vi "HILMarineTurbine.vi"() -> ()   [LabVIEW 2021]
uses:
  <vilib>/Utility/error.llb/DialogType.ctl
  <vilib>/DAQmx/read.llb/DAQmx Read (Analog 1D Wfm NChan NSamp).vi
  <vilib>/DAQmx/write.llb/DAQmx Write (Counter Frequency 1Chan 1Samp).vi
  <vilib>/Utility/file.llb/Read Delimited Spreadsheet (DBL).vi
  <vilib>/DAQmx/create/channels.llb/DAQmx Create Channel (CO-Pulse Generation-Frequency).vi
  <vilib>/DAQmx/configure/timing.llb/DAQmx Timing (Implicit).vi
  <vilib>/DAQmx/miscellaneous.llb/DAQmx Fill In Error Info.vi
  <vilib>/addons/control/pid/pid.llb/PID (DBL).vi
  <vilib>/addons/control/pid/NI_PID_pid.lvlib
panel:
  out "Waveform Graph 2":dynamicdata(graph)
  out "Waveform Graph":dynamicdata(graph)
  in  "Stop":bool
  out "XY Graph":cluster{"all rows":dbl[], "all rows":dbl[]}[](graph)
  out "Tm Turbina [Nm]":dbl
  out "Pm Turbina [W]":dbl
  in  "B [°]":dbl
  in  "Vf [m/s]":dbl
  out "Tm [Nm]":dbl
  out "Wm [RPM]":dbl
  out "P [W]":dbl
  out "IC [A]":dbl
  out "IB [A]":dbl
  out "IA [A]":dbl
  out "VCA [V]":dbl
  out "VBC [V]":dbl
  out "f [Hz] [Hz]":dbl
  out "VAB [V]":dbl
  # "Emulador de turbina marina"
  # "Voltaje"
  # "Corriente"
  # "Modelo matemático"
  # "Mediciones"
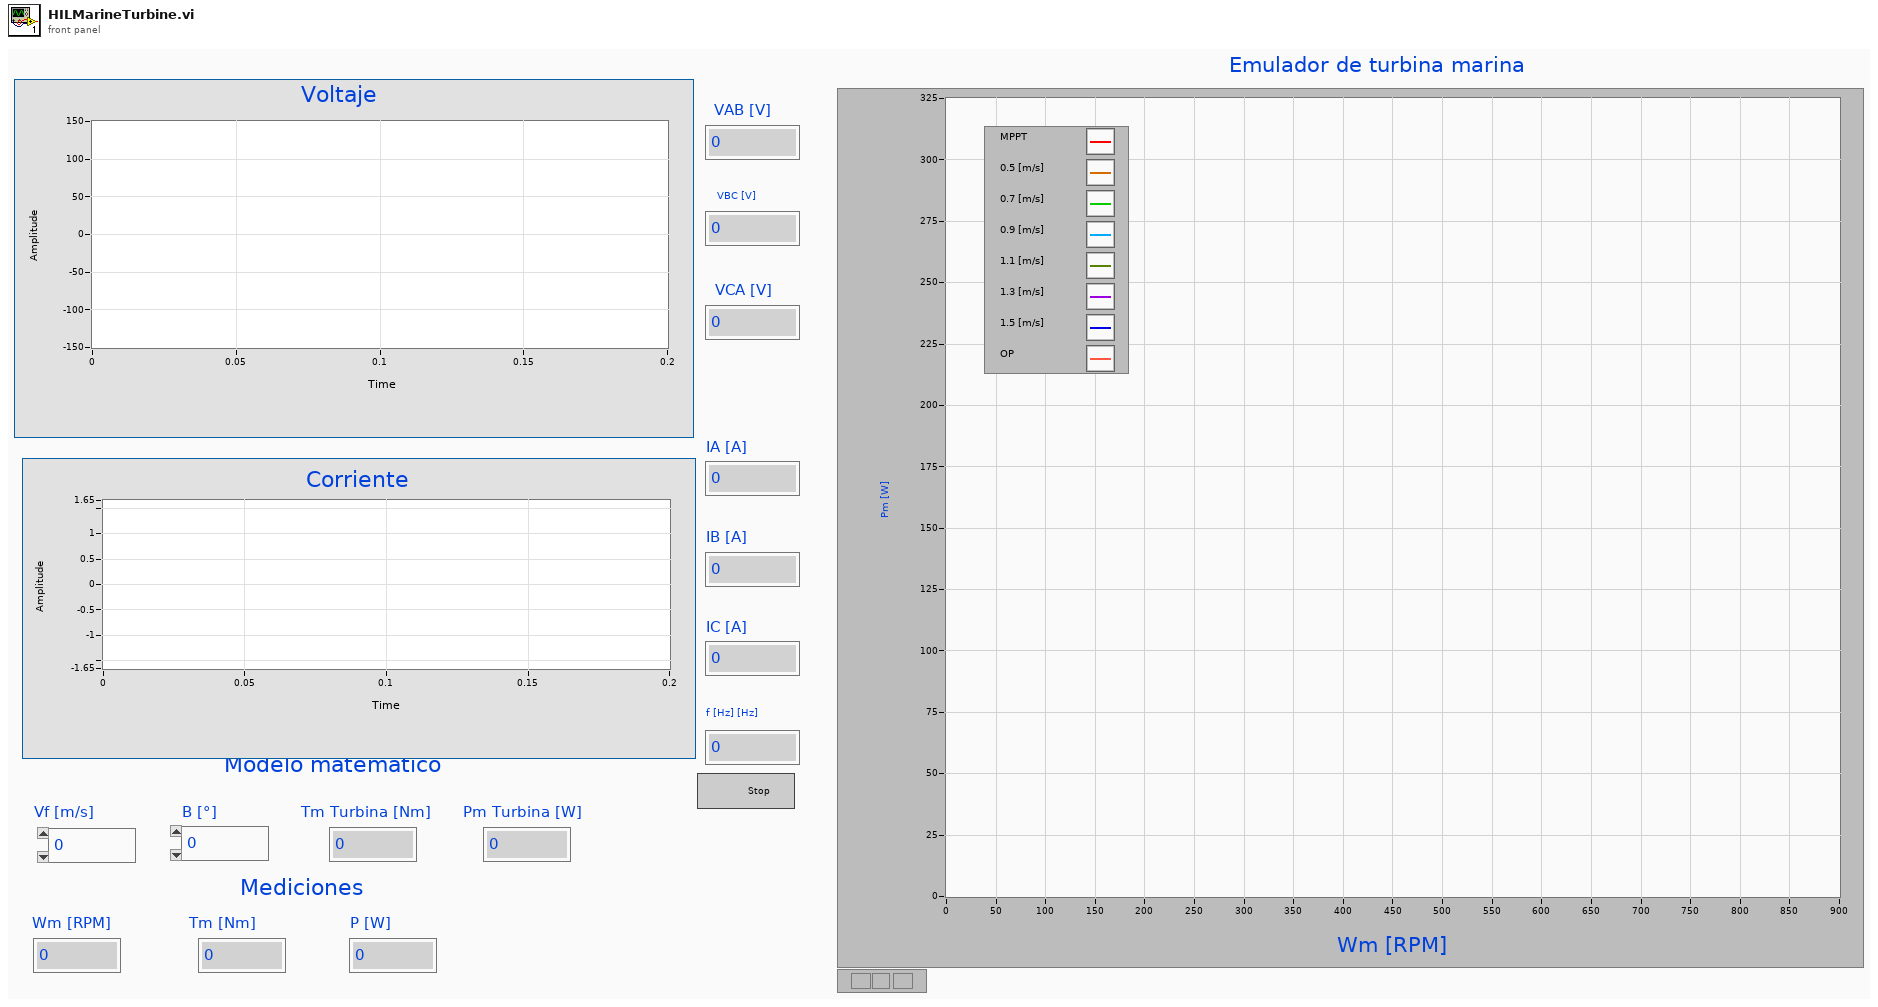
[diagram p1: front panel]
types:
  T1 = typedef "DialogType.ctl" = u16
  T2 = cluster{"proportional gain (Kc)":dbl, "integral time (Ti, min)":dbl, "derivative time (Td, min)":dbl}
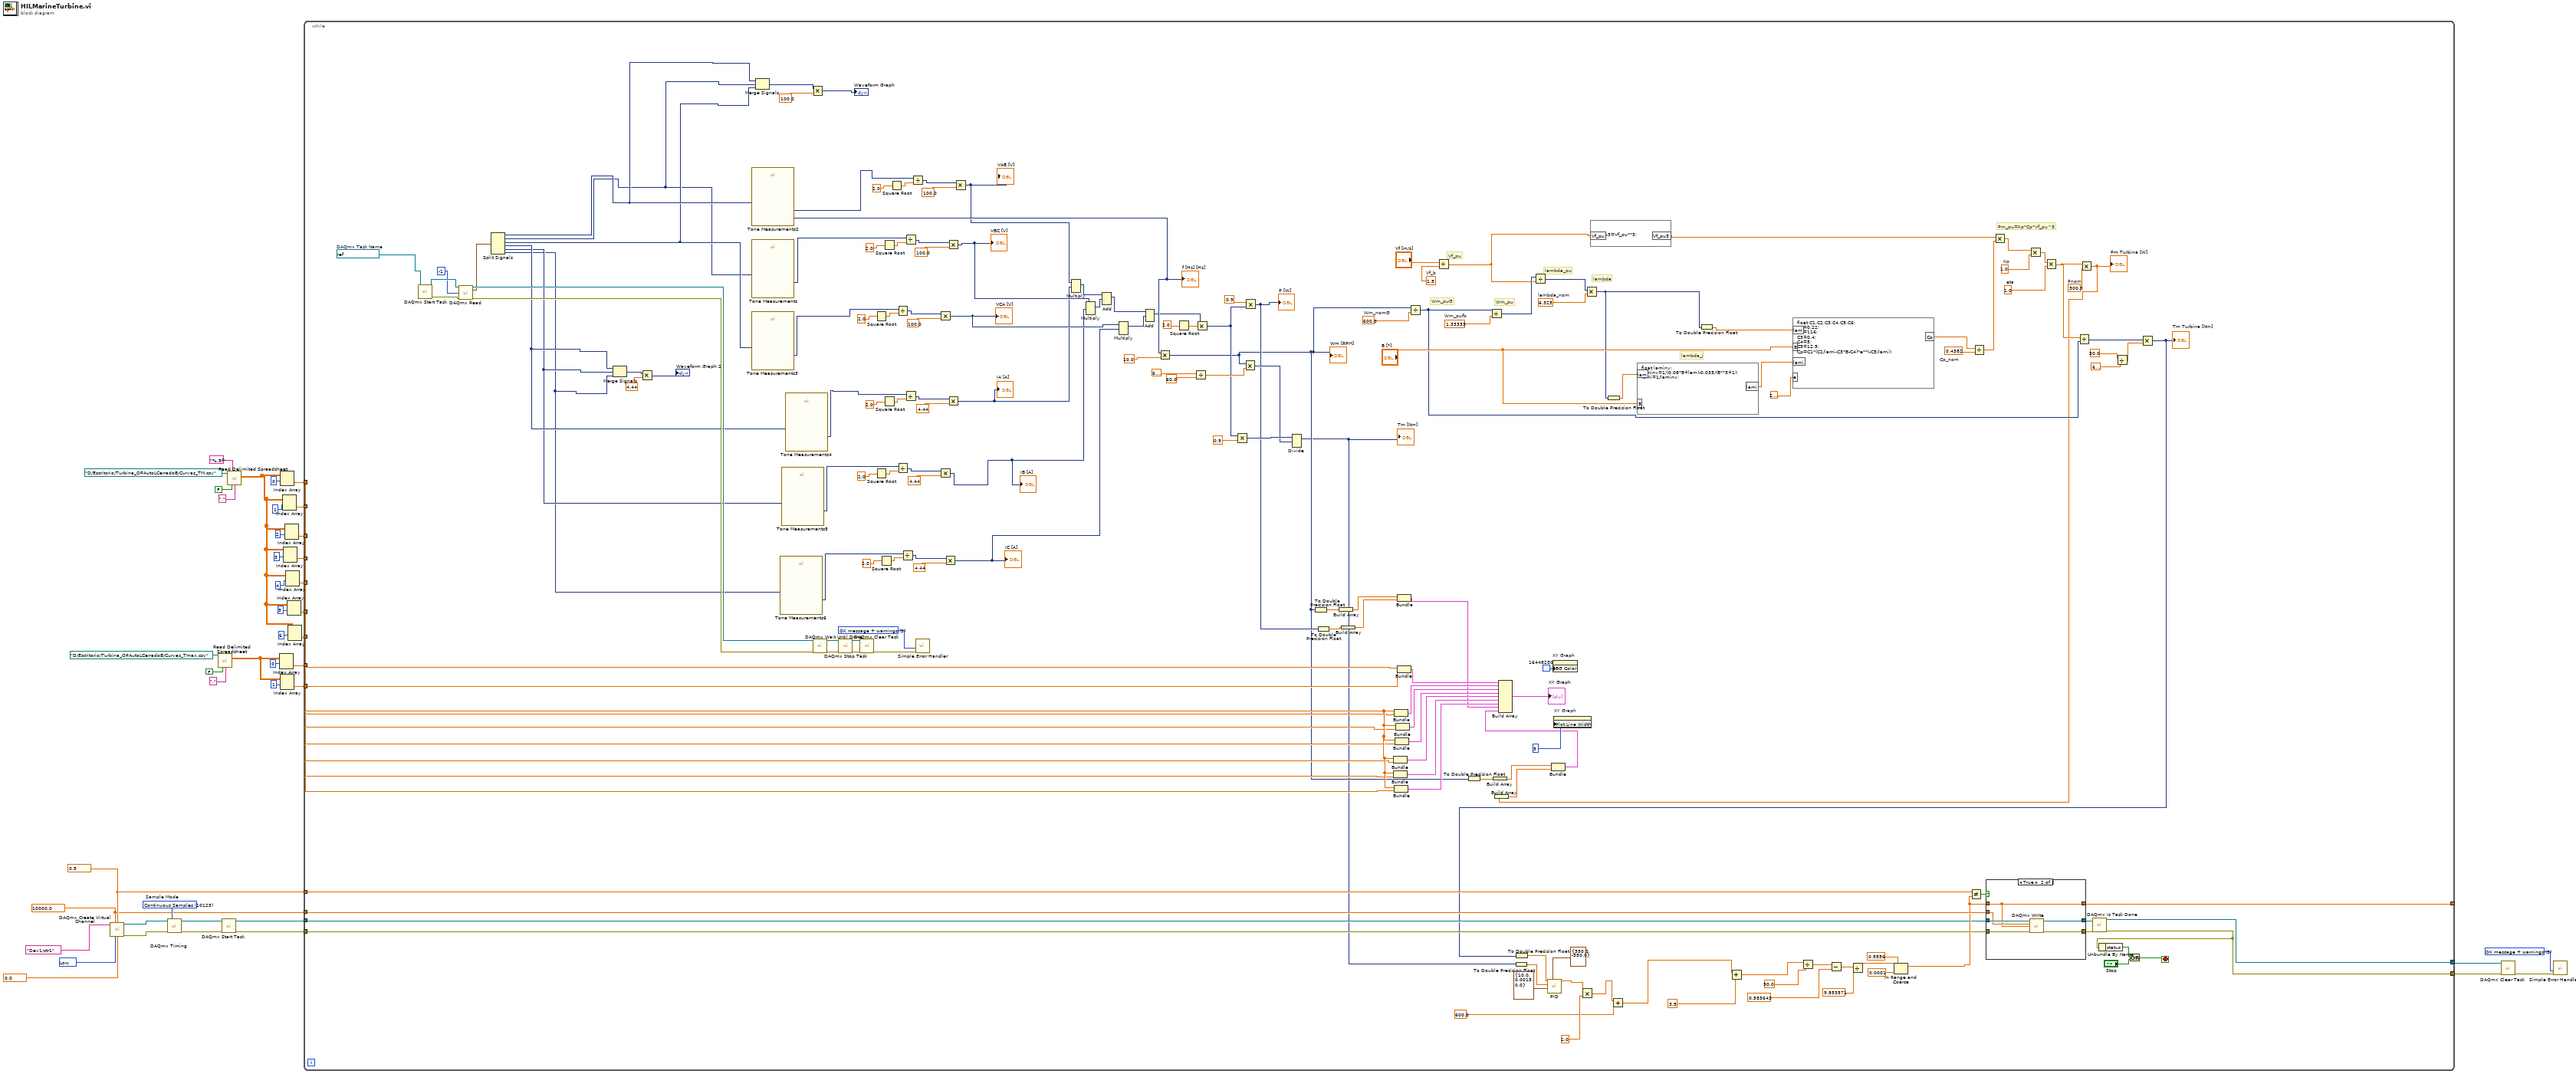
[diagram p0: block diagram]
diagram:
  w7 = T1 3 items=["no dialog", "OK message", "continue or stop message", "OK message + warnings", "continue/stop + warnings"] ("type of dialog (OK msg:1)")
  w5 = 10000.0 ("Frequency")
  w13 = 10214 items=["High"=10192, "Low"=10214] ("Idle State")
  w6 = 0.5 ("Duty Cycle")
  w16 = 10123 items=["Finite Samples"=10178, "Continuous Samples"=10123, "Hardware Timed Single Point"=12522]  # Sample Mode
  n1 = call-poly <vilib>:"DAQmx Create Virtual Channel.vi"("frequency"=w5, "duty cycle"=w6, "counter"=tag "Dev1/ctr1" ("Counter"), "idle state"=w13, "initial delay"=0.0 ("Iniital Delay")) -> ("task out"=w12:refnum<k21>, "error out"=w11:errorcluster)  [unwired: 9 in]
  n2 = call-poly <vilib>:"DAQmx Timing.vi"("task/channels in"=w12, "sample mode"=w16, "error in"=w11) -> ("task out"=w10:refnum<k21>, "error out"=w9:errorcluster)  [unwired: 11 in]
  n3 = call-poly <vilib>:"Read Delimited Spreadsheet.vi"("file path (dialog if empty)"=path "D:/Escritorio/Turbina_OPAutoLCerradoB/Curvas_Tmax.csv", "transpose? (F)"=FALSE, "delimiter (\\t)"="," ("delimiter (\\t)")) -> ("all rows"=w38:dbl[][])  [unwired: 7 in, 5 out]
  n4 = call <vilib>:"DAQmx Start Task.vi"("task/channels in"=w10, "error in"=w9) -> ("task out"=w4:refnum<k21>, "error out"=w3:errorcluster)  [unwired: 12 in]
  n5 = call-poly <vilib>:"Read Delimited Spreadsheet.vi"("file path (dialog if empty)"=path "D:/Escritorio/Turbina_OPAutoLCerradoB/Curvas_TM.csv", "format (%.3f)"="%.5f", "transpose? (F)"=FALSE, "delimiter (\\t)"="," ("delimiter (\\t)")) -> ("all rows"=w25:dbl[][])  [unwired: 6 in, 5 out]
  n6 = Index Array(array=w38, index (row)=0) -> (element=w41:dbl[])  [unwired: 1 in]
  n7 = Index Array(array=w25, index (row)=0) -> (element=w24:dbl[])  [unwired: 1 in]
  n8 = Index Array(array=w38, index (row)=1) -> (element=w37:dbl[])  [unwired: 1 in]
  n9 = Index Array(array=w25, index (row)=1) -> (element=w23:dbl[])  [unwired: 1 in]
  n10 = Index Array(array=w25, index (row)=3) -> (element=w21:dbl[])  [unwired: 1 in]
  n11 = Index Array(array=w25, index (row)=2) -> (element=w22:dbl[])  [unwired: 1 in]
  n12 = Index Array(array=w25, index (row)=4) -> (element=w20:dbl[])  [unwired: 1 in]
  n13 = Index Array(array=w25, index (row)=5) -> (element=w19:dbl[])  [unwired: 1 in]
  n14 = Index Array(array=w25, index (row)=6) -> (element=w18:dbl[])  [unwired: 1 in]
  n15 = while {
    tunnel: w41 -> [w122]
    tunnel: w37 -> [w121]
    tunnel: w24 -> [w120]
    tunnel: w23 -> [w119]
    tunnel: w22 -> [w118]
    tunnel: w21 -> [w117]
    tunnel: w20 -> [w116]
    tunnel: w19 -> [w115]
    tunnel: w18 -> [w114]
    tunnel: w6 -> [w93]
    tunnel: w5 -> [w92]
    tunnel: w4 -> [w90]
    tunnel: w3 -> [w89]
    tunnel: [w88] -> _
    tunnel: [w87] -> w2
    tunnel: [w86] -> w1
    stop <- w97 stop-if-true
    w137 = 300.0  # Pnom
    w144 = 1.0  # eta
    w146 = 1.0  # Kp
    w150 = 0.4382  # Cp_nom
    w157 = 6.325  # lambda_nom
    w158 = 1.33333  # Wm_pufb
    w160 = 1.5  # Vf_b
    w161 = 600.0  # Wm_nomG
    w205 = refnum<k21> "AI_MTurbine"  # DAQmx Task Name
    w208 = T1 3 items=["no dialog", "OK message", "continue or stop message", "OK message + warnings", "continue/stop + warnings"] ("type of dialog (OK msg:1)")
    # "Pm_pu=Kp*Cp*Vf_pu^3"
    # "lambda_i"
    # "lambda"
    # "lambda_pu"
    # "Wm_pu"
    # "Vf_pu"
    # "Wm_puG"
    n16 = call <vilib>:"DAQmx Start Task.vi"("task/channels in"=w205) -> ("task out"=w216:refnum<k21>, "error out"=w214:errorcluster)  [unwired: 13 in]
    n17 = call-poly <vilib>:"DAQmx Read.vi"("task/channels in"=w216, "number of samples per channel"=-1, "error in"=w214) -> ("task out"=w207:refnum<k21>, "data"=w204:waveform(dbl)[], "error out"=w206:errorcluster)  [unwired: 10 in]
    n18 = Split Signals(w204) -> (w55:dynamicdata, w53:dynamicdata, w54:dynamicdata, w48:dynamicdata, w47:dynamicdata, w46:dynamicdata)  [unwired: 6 in]
    n19 = Merge Signals(w48, w47, w46) -> (w45:dynamicdata)
    n20 = Multiply(x=w45, y=4.44) -> (x*y=→"Waveform Graph 2":dynamicdata)
    n21 = call "Tone Measurements3"("Signals"=w54) -> ("Amplitude"=w194:dynamicdata)  [unwired: 8 in, 2 out]
    n22 = call "Tone Measurements2"("Signals"=w55) -> ("Frequency"=w173:dynamicdata, "Amplitude"=w162:dynamicdata)  [unwired: 8 in, 1 out]
    "f [Hz] [Hz]" <- w173
    n23 = call "Tone Measurements"("Signals"=w53) -> ("Amplitude"=w199:dynamicdata)  [unwired: 8 in, 2 out]
    n24 = Merge Signals(w55, w53, w54) -> (w51:dynamicdata)
    n25 = call "Tone Measurements6"("Signals"=w46) -> ("Amplitude"=w179:dynamicdata)  [unwired: 8 in, 2 out]
    n26 = call "Tone Measurements5"("Signals"=w47) -> ("Amplitude"=w184:dynamicdata)  [unwired: 8 in, 2 out]
    n27 = call "Tone Measurements4"("Signals"=w48) -> ("Amplitude"=w189:dynamicdata)  [unwired: 8 in, 2 out]
    n28 = Multiply(x=w51, y=100.0) -> (x*y=→"Waveform Graph":dynamicdata)
    n29 = call <vilib>:"DAQmx Wait Until Done.vi"("task/channels in"=w207, "error in"=w206) -> ("task out"=w210:refnum<k21>, "error out"=w209:errorcluster)  [unwired: 12 in]
    n30 = call <vilib>:"DAQmx Stop Task.vi"("task/channels in"=w210, "error in"=w209) -> ("task out"=w212:refnum<k21>, "error out"=w211:errorcluster)  [unwired: 12 in]
    n31 = call <vilib>:"DAQmx Clear Task.vi"("task in"=w212, "error in"=w211) -> ("error out"=w213:errorcluster)  [unwired: 13 in]
    n32 = Square Root(x=2.0) -> (sqrt(x)=w198:dbl)
    n33 = Square Root(x=2.0) -> (sqrt(x)=w188:dbl)
    n34 = Square Root(x=2.0) -> (sqrt(x)=w183:dbl)
    n35 = Square Root(x=2.0) -> (sqrt(x)=w203:dbl)
    n36 = Square Root(x=2.0) -> (sqrt(x)=w193:dbl)
    n37 = Square Root(x=2.0) -> (sqrt(x)=w166:dbl)
    n38 = Divide(x=w194, y=w198) -> (x/y=w196:dynamicdata)
    n39 = Divide(x=w184, y=w188) -> (x/y=w186:dynamicdata)
    n40 = Divide(x=w179, y=w183) -> (x/y=w181:dynamicdata)
    n41 = Divide(x=w199, y=w203) -> (x/y=w201:dynamicdata)
    n42 = Divide(x=w189, y=w193) -> (x/y=w191:dynamicdata)
    n43 = Divide(x=w162, y=w166) -> (x/y=w164:dynamicdata)
    n44 = call <vilib>:"Simple Error Handler.vi"("type of dialog (OK msg:1)"=w208, "error in (no error)"=w213) -> ()  [unwired: 3 in, 5 out]
    n45 = Multiply(x=w196, y=100.0) -> (x*y=w59:dynamicdata)
    "VCA [V]" <- w59
    n46 = Multiply(x=w186, y=4.44) -> (x*y=w57:dynamicdata)
    "IB [A]" <- w57
    n47 = Multiply(x=w181, y=4.44) -> (x*y=w56:dynamicdata)
    "IC [A]" <- w56
    n48 = Multiply(x=w201, y=100.0) -> (x*y=w60:dynamicdata)
    "VBC [V]" <- w60
    n49 = Multiply(x=w191, y=4.44) -> (x*y=w58:dynamicdata)
    "IA [A]" <- w58
    n50 = Multiply(x=w164, y=100.0) -> (x*y=w61:dynamicdata)
    "VAB [V]" <- w61
    n51 = Multiply(1:w58, 2:w61) -> (0:w178:dynamicdata)  [unwired: 1 in, 1 out]
    n52 = Multiply(1:w57, 2:w60) -> (0:w177:dynamicdata)  [unwired: 1 in, 1 out]
    n53 = Add(1:w177, 2:w178) -> (0:w176:dynamicdata)  [unwired: 1 in, 1 out]
    n54 = Multiply(1:w56, 2:w59) -> (0:w175:dynamicdata)  [unwired: 1 in, 1 out]
    n55 = Add(1:w175, 2:w176) -> (0:w134:dynamicdata)  [unwired: 1 in, 1 out]
    n56 = Multiply(x=w173, y=10.0) -> (x*y=w75:dynamicdata)
    "Wm [RPM]" <- w75
    n57 = Square Root(x=2.0) -> (sqrt(x)=w135:dbl)
    n58 = Divide(x=6.283185307179586, y=60.0) -> (x/y=w168:dbl)
    n59 = Multiply(x=w134, y=w135) -> (x*y=w132:dynamicdata)
    n60 = Multiply(x=w132, y=0.9) -> (x*y=w171:dynamicdata)
    n61 = Multiply(x=w75, y=w168) -> (x*y=w167:dynamicdata)
    n62 = Multiply(x=0.9, y=w132) -> (x*y=w127:dynamicdata)
    "P [W]" <- w127
    n63 = Divide(1:w167, 2:w171) -> (0:w66:dynamicdata)  [unwired: 1 in, 1 out]
    "Tm [Nm]" <- w66
    n64 = To Double Precision Float(number=w75) -> (double precision float=w126:dbl)
    n65 = To Double Precision Float(number=w127) -> (double precision float=w125:dbl)
    n66 = Build Array(w126) -> (w124:dbl[])
    n67 = Build Array(w125) -> (w123:dbl[])
    n68 = Bundle("all rows"=w120, "all rows"=w115) -> (w108:cluster{"all rows":dbl[], "all rows":dbl[]})  [unwired: 1 in]
    n69 = Bundle("all rows"=w120, "all rows"=w116) -> (w109:cluster{"all rows":dbl[], "all rows":dbl[]})  [unwired: 1 in]
    n70 = Bundle("all rows"=w120, "all rows"=w119) -> (w112:cluster{"all rows":dbl[], "all rows":dbl[]})  [unwired: 1 in]
    n71 = Bundle("all rows"=w120, "all rows"=w114) -> (w107:cluster{"all rows":dbl[], "all rows":dbl[]})  [unwired: 1 in]
    n72 = Bundle("all rows"=w120, "all rows"=w117) -> (w110:cluster{"all rows":dbl[], "all rows":dbl[]})  [unwired: 1 in]
    n73 = Bundle("all rows"=w120, "all rows"=w118) -> (w111:cluster{"all rows":dbl[], "all rows":dbl[]})  [unwired: 1 in]
    n74 = Bundle("all rows"=w122, "all rows"=w121) -> (w113:cluster{"all rows":dbl[], "all rows":dbl[]})  [unwired: 1 in]
    n75 = Bundle(w124, w123) -> (w106:cluster{dbl[], dbl[]})  [unwired: 1 in]
    n76 = Divide(x=w75, y=w161) -> (x/y=w141:dynamicdata)
    n77 = Divide(x="Vf [m/s]", y=w160) -> (x/y=w140:dbl)
    n78 = To Double Precision Float(number=w75) -> (double precision float=w78:dbl)
    n79 = Divide(x=w141, y=w158) -> (x/y=w142:dynamicdata)
    n80 = Build Array(w78) -> (w77:dbl[])
    n81 = To Double Precision Float(number=w66) -> (double precision float=w71:dbl)
    n82 = Divide(x=w142, y=w140) -> (x/y=w156:dynamicdata)
    n83 = property on="XY Graph" class="XYGraph (strict)"("BG Color"=u32 16448250 ("Plot Area:Colors:BG Color")) -> ()  [unwired: 2 in, 2 out]
    n84 = property on="XY Graph" class="XYGraph (strict)"("Plot.Line Width"=u8 5) -> ()  [unwired: 2 in, 2 out]
    n85 = Multiply(x=w156, y=w157) -> (x*y=w151:dynamicdata)
    n86 = formula code="Vf_pu3=Vf_pu**3;"("Vf_pu"=w140) -> ("Vf_pu3"=w139:dbl)
    n87 = To Double Precision Float(number=w151) -> (double precision float=w155:dbl)
    n88 = formula code="float laminv;\nlaminv=1/(0.08*B+lam)-0.035/(B**3+1);\nlami=1/laminv;"("lam"=w155, "B"="B [°]") -> ("lami"=w154:dbl)
    n89 = To Double Precision Float(number=w151) -> (double precision float=w152:dbl)
    n90 = formula code="float C1,C2,C3,C4,C5,C6;\nC1=0.22;\nC2=116;\nC3=0.4;\nC4=5;\nC5=12.5;\nCp=C1*(C2/lami-C3*B-C4)*e**(-C5/lami);"("lam"=w152, "B"="B [°]", "lami"=w154, "e"=2.718281828459045) -> ("Cp"=w149:dbl)
    n91 = Divide(x=w149, y=w150) -> (x/y=w148:dbl)
    n92 = Multiply(x=w139, y=w148) -> (x*y=w147:dbl)
    n93 = Multiply(x=w147, y=w146) -> (x*y=w145:dbl)
    n94 = Multiply(x=w145, y=w144) -> (x*y=w138:dbl)
    n95 = Divide(x=w138, y=w141) -> (x/y=w129:dynamicdata)
    n96 = Multiply(x=w138, y=w137) -> (x*y=w74:dbl)
    "Pm Turbina [W]" <- w74
    n97 = Build Array(w74) -> (w76:dbl[])
    n98 = Bundle(w77, w76) -> (w73:cluster{dbl[], dbl[]})  [unwired: 1 in]
    n99 = Build Array(w113, w112, w111, w110, w109, w108, w107, w106, w73) -> (→"XY Graph":cluster{"all rows":dbl[], "all rows":dbl[]}[])
    n100 = Divide(x=30.0, y=6.283185307179586) -> (x/y=w128:dbl)
    n101 = Multiply(x=w129, y=w128) -> (x*y=w67:dynamicdata)
    "Tm Turbina [Nm]" <- w67
    n102 = To Double Precision Float(number=w67) -> (double precision float=w70:dbl)
    n103 = call-poly <vilib>:"PID.vi"("output range"=cluster{"output high":dbl, "output low":dbl} {"output high"=350.0, "output low"=-350.0}, "PID gains"=T2 {"proportional gain (Kc)"=10.0, "integral time (Ti, min)"=0.0015, "derivative time (Td, min)"=0.0}, "process variable"=w71, "setpoint"=w70) -> ("output"=w68:dbl)  [unwired: 6 in, 1 out]
    n104 = Multiply(x=w68, y=1.0 ("signo")) -> (x*y=w63:dbl)
    n105 = Add(x=w63, y=600.0 ("Numeric 3")) -> (x+y=w65:dbl)
    n106 = Add(x=w65, y=3.5 ("Numeric")) -> (x+y=w79:dbl)
    n107 = Divide(x=w79, y=90.0) -> (x/y=w85:dbl)
    n108 = Subtract(x=w85, y=0.583643) -> (x-y=w84:dbl)
    n109 = Divide(x=w84, y=9.853571) -> (x/y=w83:dbl)
    n110 = In Range and Coerce(upper limit=0.9556, x=w83, lower limit=0.0001) -> (coerced(x)=w91:dbl)  [unwired: 1 out]
    n111 = Not Equal?(x=w93, y=w91) -> (x != y?=w98:bool)
    n112 = case shown="True" w98 {
      tunnel: w89 -> [w217 w225]
      tunnel: w90 -> [w218 w224]
      tunnel: [w218 w223] -> w100
      tunnel: [w217 w222] -> w99
      tunnel: w91 -> [w219 w220]
      tunnel: w92 -> [_ w221]
      tunnel: [w219 w220] -> w88
      frame False {
      }
      frame True {
        n113 = call-poly <vilib>:"DAQmx Write.vi"("task/channels in"=w224, "frequency"=w221, "duty cycle"=w220, "error in"=w225) -> ("task out"=w223:refnum<k21>, "error out"=w222:errorcluster)  [unwired: 9 in, 1 out]
      }
    }
    n114 = call <vilib>:"DAQmx Is Task Done.vi"("task/channels in"=w100, "error in"=w99) -> ("task out"=w87:refnum<k21>, "error out"=w86:errorcluster)  [unwired: 11 in, 1 out]
    n115 = Unbundle By Name(w86) -> ("status"=w102:bool)
    n116 = Or(x=w102, y="Stop") -> (x .or. y?=w97:bool)
  }
  n117 = call <vilib>:"DAQmx Clear Task.vi"("task in"=w2, "error in"=w1) -> ("error out"=w8:errorcluster)  [unwired: 13 in]
  n118 = call <vilib>:"Simple Error Handler.vi"("type of dialog (OK msg:1)"=w7, "error in (no error)"=w8) -> ()  [unwired: 3 in, 5 out]
